vi "enable control.vi"(8 "error in (no error)":errorcluster, 10 "enabled? (T)":bool=TRUE, 11 "control in":refnum<vi>) -> (0 "error out":errorcluster, 2 "enabled out":bool=TRUE, 3 "control out":refnum<vi>)   [LabVIEW 2014, in "Shared Memory editor node.lvclass"]
uses:
  Shared Memory editor node.lvclass
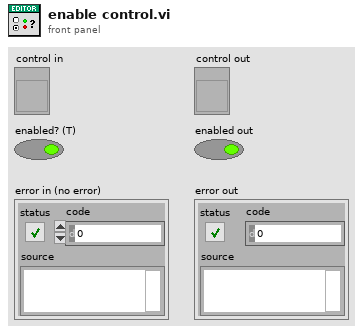
[diagram p1: front panel]
types:
  T1 = enum8{"Enabled", "Disabled", "Disabled and Grayed Out"}
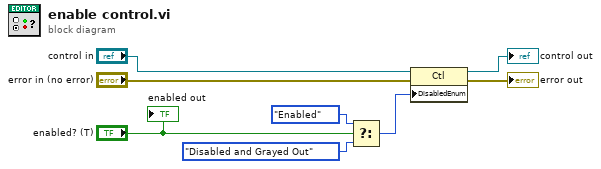
[diagram p0: block diagram]
diagram:
  n1 = Select(t=T1."Enabled" ("Disabled"), s="enabled? (T)", f=T1."Disabled and Grayed Out" ("Disabled")) -> (s? t:f=w8:T1)
  n2 = property class="Ctl"(reference="control in", error in="error in (no error)", "DisabledEnum"=w8) -> (reference out=→"control out":refnum<vi>, error out=→"error out":errorcluster)
  "enabled out" <- "enabled? (T)"
